vi "Balance_Sweep_Multi.vi"() -> ()   [LabVIEW 2011]
panel:
  out "Current Mode":bool
  out "Current Measurement Time (ms)":u32
  out "Current Stop Angle (deg)":dbl
  out "Current Filename":string
  out "error out":errorcluster
  in  "Sweep Cluster Array":T1(array[cluster])=[{"Filename"="27ms_SJ_OFF_4_n2", "Stop Angle (deg)"=-2.0, "Sample Freq (Hz)"=20000.0, "Measurement Time (ms)"=0, "Mode"=FALSE}, {"Filename"="27ms_SJ_OFF_n2_n8", "Stop Angle (deg)"=-8.0, "Sample Freq (Hz)"=20000.0, "Measurement Time (ms)"=0, "Mode"=FALSE}, {"Filename"="27ms_SJ_OFF_n8_n14", "Stop Angle (deg)"=-14.0, "Sample Freq (Hz)"=20000.0, "Measurement Time (ms)"=0, "Mode"=FALSE}, {"Filename"="27ms_SJ_OFF_n14_n20", "Stop Angle (deg)"=-20.0, "Sample Freq (Hz)"=20000.0, "Measurement Time (ms)"=0, "Mode"=FALSE}, {"Filename"="27ms_SJ_OFF_n20_n24", "Stop Angle (deg)"=-24.0, "Sample Freq (Hz)"=20000.0, "Measurement Time (ms)"=0, "Mode"=FALSE}, {"Filename"="27ms_SJ_OFF_n24_n20", "Stop Angle (deg)"=-20.0, "Sample Freq (Hz)"=20000.0, "Measurement Time (ms)"=0, "Mode"=FALSE}, {"Filename"="27ms_SJ_OFF_n20_n14", "Stop Angle (deg)"=-14.0, "Sample Freq (Hz)"=20000.0, "Measurement Time (ms)"=0, "Mode"=FALSE}, {"Filename"="27ms_SJ_OFF_n14_n8", "Stop Angle (deg)"=-8.0, "Sample Freq (Hz)"=20000.0, "Measurement Time (ms)"=0, "Mode"=FALSE}, {"Filename"="27ms_SJ_OFF_n14_n8", "Stop Angle (deg)"=-2.0, "Sample Freq (Hz)"=20000.0, "Measurement Time (ms)"=0, "Mode"=FALSE}]
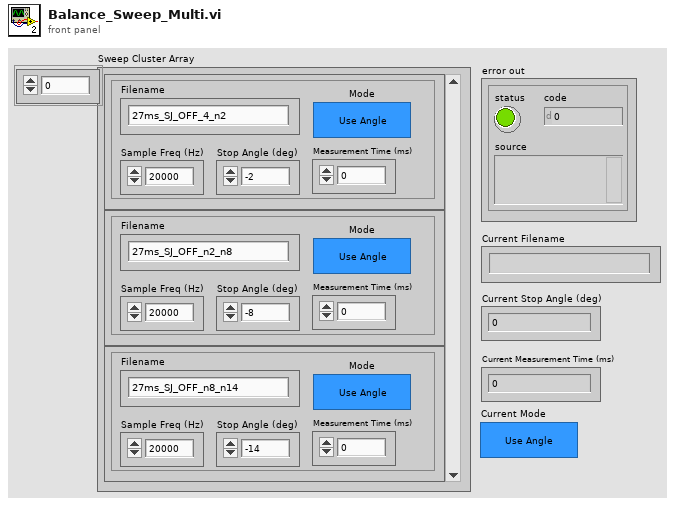
[diagram p1: front panel]
types:
  T1 = cluster{"Filename":string, "Stop Angle (deg)":dbl, "Sample Freq (Hz)":dbl, "Measurement Time (ms)":u32, "Mode":bool}[]
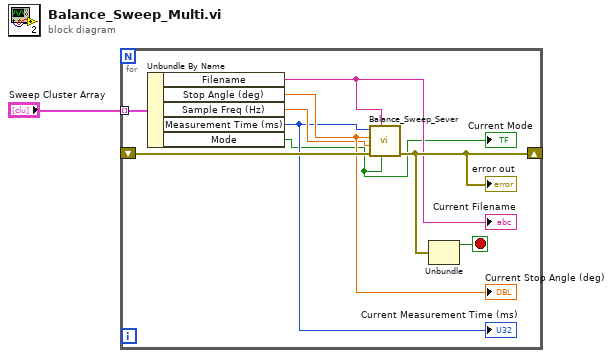
[diagram p0: block diagram]
diagram:
  n1 = for {
    shift-right: [w9] -> _
    shift-left: _ -> [w8]
    tunnel: "Sweep Cluster Array" -> [w7] mode=indexing
    stop <- w10 stop-if-true
    n2 = Unbundle By Name(w7) -> ("Filename"=w4:string, "Stop Angle (deg)"=w6:dbl, "Sample Freq (Hz)"=w5:dbl, "Measurement Time (ms)"=w3:u32, "Mode"=w2:bool)
    "Current Filename" <- w4
    "Current Stop Angle (deg)" <- w6
    "Current Measurement Time (ms)" <- w3
    "Current Mode" <- w2
    n3 = call "Balance_Sweep_Sever.vi"("Mode"=w2, "Filename"=w4, "error in"=w8, "Sample Freq (Hz)"=w5, "Stop Angle (deg)"=w6, "Measurement Time (ms)"=w3) -> ("error out"=w9:errorcluster)  [unwired: 5 in]
    "error out" <- w9
    n4 = Unbundle(w9) -> ("status"=w10:bool)  [unwired: 2 out]
  }
